vi "IVCurveFit.vi"(11 "IVData":dbl[][](array[numeric])) -> (1 "best fit parameters":dbl[](array[numeric]), 2 "Conductance":dbl, 3 "Capacitance":dbl)   [LabVIEW 2020]
uses:
  <vilib>/Analysis/6fits.llb/Curve Fitting Criteria.ctl
  <vilib>/gmath/NumericalOptimization/Nonlinear Curve Fit LM formula string.vi
  <vilib>/Analysis/NI_AALPro.lvlib
  <vilib>/gmath/NI_Gmath.lvlib
panel:
  out "XY Graph":cluster{dbl[], dbl[]}[](graph)
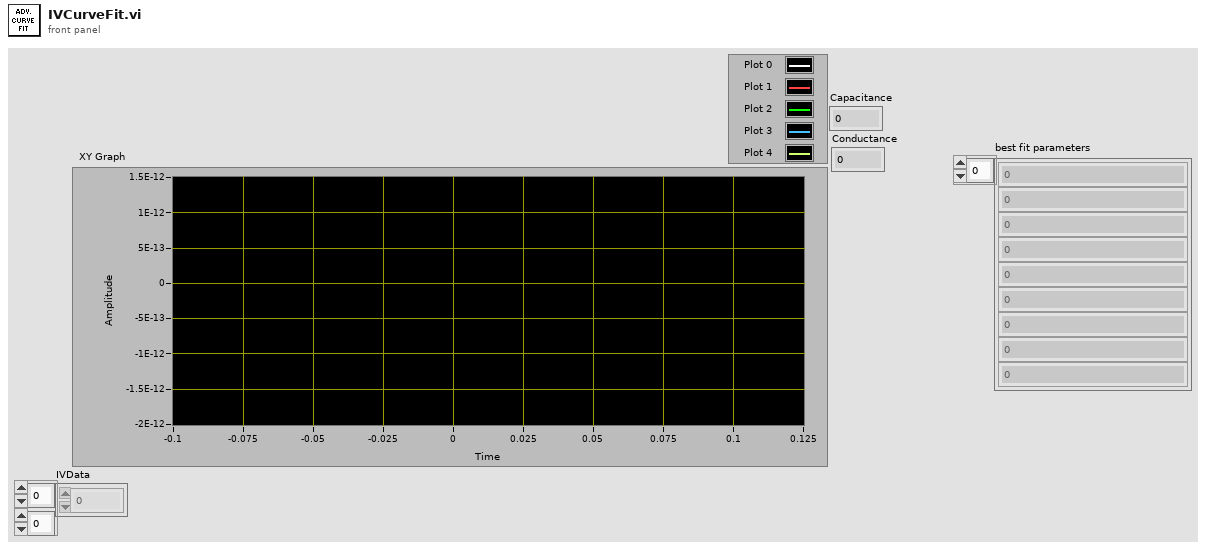
[diagram p1: front panel]
types:
  T1 = cluster{"model":string, "Parameters":string[], "x":string}
  T2 = cluster{"Conductance":i32, "Intercept":i32, "Voltage0":i32, "ChargeCapacitance":i32}
  T3 = typedef "NI_AALPro.lvlib/Curve Fitting Criteria.ctl" = u16
  T4 = cluster{"IVData":dbl[], "best nonlinear fit":dbl[]}[]
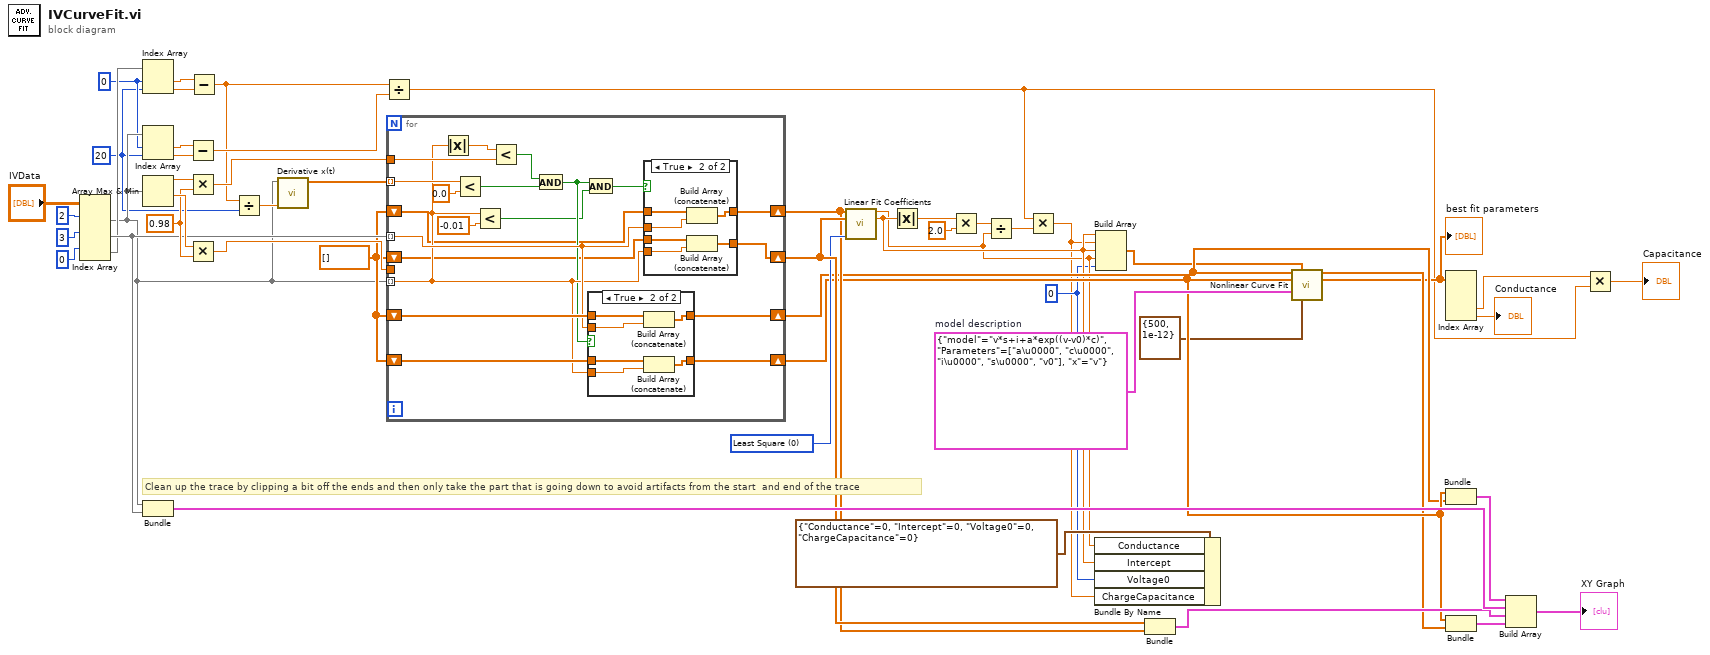
[diagram p0: block diagram]
diagram:
  w11 = 20 ("index")
  w12 = 0 ("index")
  w20 = 0
  w30 = T1 {"model"="v*s+i+a*exp((v-v0)*c)", "Parameters"=["a\u0000", "c\u0000", "i\u0000", "s\u0000", "v0"], "x"="v"}  # model description
  w37 = T3 0 items=["Least Square", "Least Absolute Residual", "Bisquare"] ("method")
  w40 = dbl[] []
  w48 = 0.98
  # "Clean up the trace by clipping a bit off the ends and then only take the part that is going down to avoid artifacts from the start  and end of the trace"
  n1 = Index Array(array="IVData", index (row) #1=2 ("index (row)"), index (row) #2=3 ("index (row)"), index (row) #3=0 ("index (row)")) -> (element #1=w13:dbl[], element #2=w44:dbl[], element #3=w17:dbl[])  [unwired: 3 in]
  n2 = Index Array(array=w17, index #1=w12, index #2=w11) -> (element #1=w16:dbl, element #2=w15:dbl)
  n3 = Index Array(array=w13, index #1=w12, index #2=w11) -> (element #1=w10:dbl, element #2=w9:dbl)
  n4 = Array Max & Min(array=w13) -> (max value=w51:dbl, min value=w50:dbl)  [unwired: 2 out]
  n5 = Bundle("IVData"=w13, "IVData"=w44) -> (w42:cluster{"IVData":dbl[], "IVData":dbl[]})  [unwired: 1 in]
  n6 = Subtract(x=w10, y=w9) -> (x-y=w8:dbl)
  n7 = Multiply(x=w51, y=w48) -> (x*y=w22:dbl)
  n8 = Multiply(x=w50, y=w48) -> (x*y=w49:dbl)
  n9 = Subtract(x=w16, y=w15) -> (x-y=w7:dbl)
  n10 = Divide(x=w7, y=w11) -> (x/y=w14:dbl)
  n11 = call <vilib>:"Derivative x(t).vi"("dt"=w14, "X"=w13) -> ("dX/dt"=w41:dbl[])  [unwired: 8 in, 1 out]
  n12 = Divide(x=w7, y=w8) -> (x/y=w1:dbl)
  n13 = for {
    tunnel: w22 -> [w68]
    tunnel: w49 -> [_]
    tunnel: w13 -> [w58] mode=indexing
    tunnel: w44 -> [w59] mode=indexing
    shift-right: [w71] -> w29
    shift-left: w40 -> [w61]
    shift-right: [w70] -> w28
    shift-left: w40 -> [w60]
    tunnel: w41 -> [w66] mode=indexing
    shift-right: [w63] -> w38
    shift-left: w40 -> [w53]
    shift-right: [w62] -> w36
    shift-left: w40 -> [w52]
    n14 = Absolute Value(x=w58) -> (abs(x)=w69:dbl)
    n15 = Less?(x=w66, y=0.0) -> (x < y?=w64:bool)
    n16 = Less?(x=w58, y=-0.01) -> (x < y?=w55:bool)
    n17 = Less?(x=w69, y=w68) -> (x < y?=w67:bool)
    n18 = And(x=w67, y=w64) -> (x .and. y?=w56:bool)
    n19 = And(x=w56, y=w55) -> (x .and. y?=w54:bool)
    n20 = case shown="True" w56 {
      tunnel: w61 -> [w81 w87]
      tunnel: w60 -> [w80 w86]
      tunnel: [w81 w85] -> w71
      tunnel: [w80 w84] -> w70
      tunnel: w58 -> [_ w83]
      tunnel: w59 -> [_ w82]
      frame False {
      }
      frame True {
        n21 = Build Array (concatenate)(w86, w82) -> (w84:dbl[])
        n22 = Build Array (concatenate)(w87, w83) -> (w85:dbl[])
      }
    }
    n23 = case shown="True" w54 {
      tunnel: w53 -> [w73 w79]
      tunnel: w52 -> [w72 w78]
      tunnel: [w73 w77] -> w63
      tunnel: [w72 w76] -> w62
      tunnel: w58 -> [_ w75]
      tunnel: w59 -> [_ w74]
      frame False {
      }
      frame True {
        n24 = Build Array (concatenate)(w78, w74) -> (w76:dbl[])
        n25 = Build Array (concatenate)(w79, w75) -> (w77:dbl[])
      }
    }
  }
  n26 = call <vilib>:"Linear Fit Coefficients.vi"("Y"=w36, "X"=w38, "method"=w37) -> ("slope"=w23:dbl, "intercept"=w24:dbl)  [unwired: 10 in, 1 out]
  n27 = Absolute Value(x=w24) -> (abs(x)=w34:dbl)
  n28 = Multiply(x=w34, y=2.0) -> (x*y=w32:dbl)
  n29 = Divide(x=w32, y=w23) -> (x/y=w31:dbl)
  n30 = Multiply(x=w1, y=w31) -> (x*y=w6:dbl)
  n31 = Bundle By Name(cluster=T2 {"Conductance"=0, "Intercept"=0, "Voltage0"=0, "ChargeCapacitance"=0} ("input cluster"), "Conductance"=w23, "Intercept"=w24, "Voltage0"=w20, "ChargeCapacitance"=w6) -> ()  [unwired: 1 out]
  n32 = Build Array(w24, w6, w24, w23, w20) -> (w25:dbl[])
  n33 = Bundle(w38, w36) -> (w39:cluster{dbl[], dbl[]})  [unwired: 1 in]
  n34 = call-poly <vilib>:"Nonlinear Curve Fit.vi"("Y"=w28, "initial parameters"=w25, "X"=w29, "model description"=w30, "termination"=cluster{"max iteration":i32, "tolerance":dbl} {"max iteration"=500, "tolerance"=1e-12}) -> ("best nonlinear fit"=w27:dbl[], "best fit parameters"=w5:dbl[])  [unwired: 6 in, 3 out]
  "best fit parameters" <- w5
  n35 = Index Array(array=w5) -> (element #3=w4:dbl, element #4=→"Conductance":dbl)  [unwired: 4 in, 2 out]
  n36 = Bundle(w29, w28) -> (w43:cluster{dbl[], dbl[]})  [unwired: 1 in]
  n37 = Bundle(w29, "best nonlinear fit"=w27) -> (w26:cluster{dbl[], "best nonlinear fit":dbl[]})  [unwired: 1 in]
  n38 = Build Array(w43, w42, w39, w26) -> (→"XY Graph":T4)
  n39 = Multiply(x=w4, y=w1) -> (x*y=→"Capacitance":dbl)
